vi "QTrkGetDerivedSettings.vi"(8 "error in (no error)":errorcluster, 11 "QTrk Instance":T3) -> (0 "error out":errorcluster, 1 "ZLUT Radial Steps":i32, 2 "Derived settings":T1={"QTrk Settings"={"Image width"=150, "Image height"=150, "Number of threads (CPU based)"=-1, "CUDA Device"=-2, "COM Background correction factor"=0.0, "ZLUT MinRadius"=8.0, "ZLUT Radial sample density"=5.0, "ZLUT Angular sample density"=2.0, "ZLUT ROI Coverage"=0.7, "QI Iterations"=2, "QI MinRadius"=5.0, "QI Radial sample density"=2.0, "QI Angular sample density"=0.7, "QI ROI Coverage"=1.0, "QI Angular Step \nIteration Factor"=128.0, "XCOR Profile Length"=32, "XCOR Profile Width"=2, "XCOR Iterations"=1, "Gaussian 2D Fit Iterations"=2, "Gaussian 2D Sigma (pixels)"=3.0}, "Derived settings"={"ZLUT Radial Steps"=0, "ZLUT Angular Steps"=0, "ZLUT Max Radius"=0.0, "QI Radial Steps"=0, "QI Angular Steps\nPer Quadrant"=0, "QI Max Radius"=0.0}}, 3 "QTrk Instance (out)":T3, 4 "ZLUT Max Radius":sgl, 6 "ROI size":cluster{"Image width":i32, "Image height":i32})   [LabVIEW 2011]
uses:
  QTrkInstance.ctl
  QTrkComputedSettings.ctl
  QTrkSettings.ctl
  QTrkDLL.vi
panel:
  # "-2: Use all devices\n-1: Use best device"
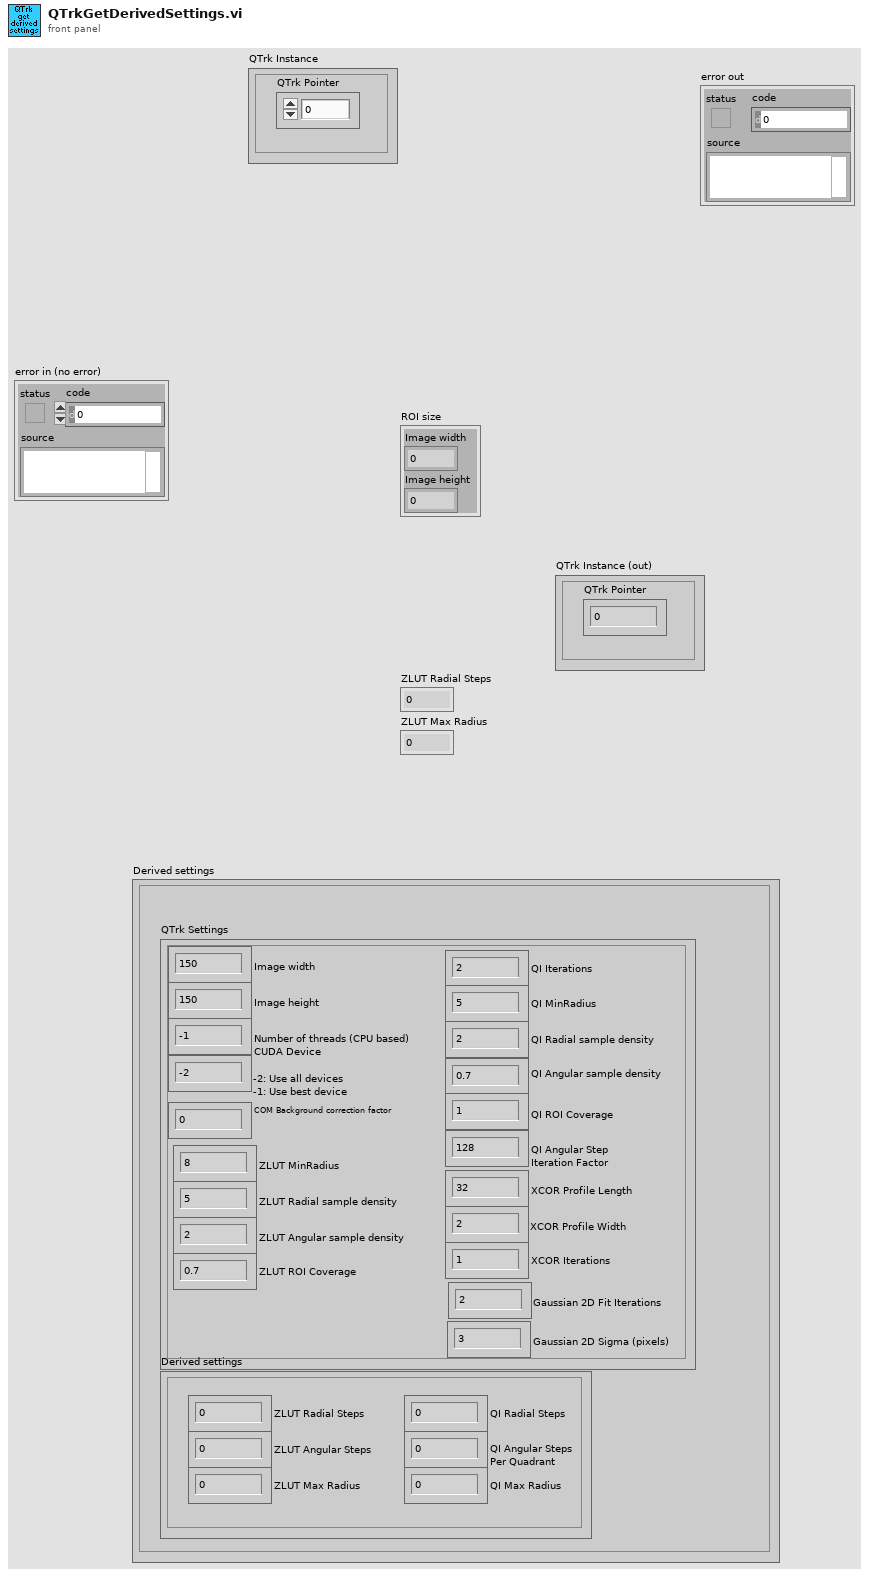
[diagram p1: front panel]
types:
  T1 = typedef "QTrkComputedSettings.ctl" = cluster{"QTrk Settings":T2, "Derived settings":cluster{"ZLUT Radial Steps":i32, "ZLUT Angular Steps":i32, "ZLUT Max Radius":sgl, "QI Radial Steps":i32, "QI Angular Steps\nPer Quadrant":i32, "QI Max Radius":sgl}}
  T2 = typedef "QTrkSettings.ctl" = cluster{"Image width":i32, "Image height":i32, "Number of threads (CPU based)":i32, "CUDA Device":i32, "COM Background correction factor":sgl, "ZLUT MinRadius":sgl, "ZLUT Radial sample density":sgl, "ZLUT Angular sample density":sgl, "ZLUT ROI Coverage":sgl, "QI Iterations":i32, "QI MinRadius":sgl, "QI Radial sample density":sgl, "QI Angular sample density":sgl, "QI ROI Coverage":sgl, "QI Angular Step \nIteration Factor":sgl, "XCOR Profile Length":i32, "XCOR Profile Width":i32, "XCOR Iterations":i32, "Gaussian 2D Fit Iterations":i32, "Gaussian 2D Sigma (pixels)":sgl}
  T3 = typedef "QTrkInstance.ctl" = cluster{"QTrk Pointer":u64}
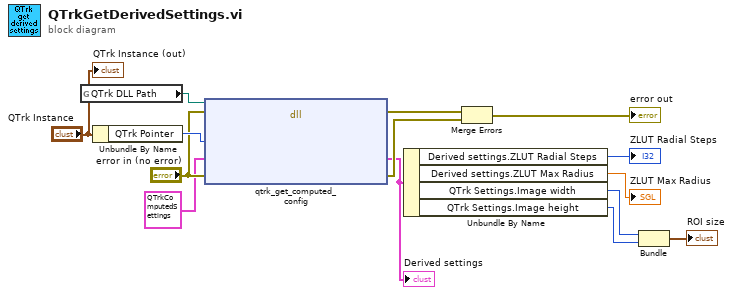
[diagram p0: block diagram]
diagram:
  n1 = global read "QTrkDLL.vi" "QTrk DLL Path"() -> (w12:path)
  n2 = Unbundle By Name("QTrk Instance") -> ("QTrk Pointer"=w13:u64)
  n3 = dll-call lib="D:/jcnossen1/cudaqi-tracker/bin/jtrk-labview.dll" fn="qtrk_get_computed_config"(path in=w12, error in="error in (no error)", "tracker"=w13, "config"=T1 {"QTrk Settings"={"Image width"=150, "Image height"=150, "Number of threads (CPU based)"=-1, "CUDA Device"=-2, "COM Background correction factor"=0.0, "ZLUT MinRadius"=8.0, "ZLUT Radial sample density"=5.0, "ZLUT Angular sample density"=2.0, "ZLUT ROI Coverage"=0.7, "QI Iterations"=2, "QI MinRadius"=5.0, "QI Radial sample density"=2.0, "QI Angular sample density"=0.7, "QI ROI Coverage"=1.0, "QI Angular Step \nIteration Factor"=128.0, "XCOR Profile Length"=32, "XCOR Profile Width"=2, "XCOR Iterations"=1, "Gaussian 2D Fit Iterations"=0, "Gaussian 2D Sigma (pixels)"=0.0}, "Derived settings"={"ZLUT Radial Steps"=0, "ZLUT Angular Steps"=0, "ZLUT Max Radius"=0.0, "QI Radial Steps"=0, "QI Angular Steps\nPer Quadrant"=0, "QI Max Radius"=0.0}} ("QTrk Computed Settings"), "error"="error in (no error)") -> (error out=w10:errorcluster, "config"=w6:T1, "error"=w9:errorcluster)  [unwired: 3 in, 1 out]
  "Derived settings" <- w6
  n4 = Unbundle By Name(w6) -> ("Derived settings.ZLUT Radial Steps"=→"ZLUT Radial Steps":i32, "Derived settings.ZLUT Max Radius"=→"ZLUT Max Radius":sgl, "QTrk Settings.Image width"=w3:i32, "QTrk Settings.Image height"=w2:i32)
  n5 = Merge Errors(w10, w9) -> (→"error out":errorcluster)
  n6 = Bundle("Image width"=w3, "Image height"=w2) -> (→"ROI size":cluster{"Image width":i32, "Image height":i32})  [unwired: 1 in]
  "QTrk Instance (out)" <- "QTrk Instance"
